vi "Station References Global.vi"() -> ()   [LabVIEW 2018]
panel:
  in  "Run Cal Popup":bool
  out "Oven_RTL":bool
  out "DMM3_RTL":bool
  out "DMM2_RTL":bool
  out "DMM1_RTL":bool
  out "PS3_RTL":bool
  out "PS2_RTL":bool
  out "PS1_RTL":bool
  out "RF Switch_RTL":bool
  out "NFA_RTL":bool
  out "SigGen3_RTL":bool
  out "SigGen2_RTL":bool
  out "SigGen1_RTL":bool
  out "SA_RTL":bool
  out "PNA_RTL":bool
  out "VNA_RTL":bool
  in  "Gantry":refnum<visa-resource-name>="GPIB0::9::INSTR"
  out "Gantry Model":string
  out "Gantry Present?":bool
  in  "RF Switch":refnum<visa-resource-name>="GPIB0::9::INSTR"
  out "RF Switch Model":string
  out "RF Switch Present?":bool
  out "PNA Model":string
  in  "PNA":refnum<visa-resource-name>
  out "PNA Present?":bool
  out "TempSense1":tag
  out "TempSense1 Model":string
  out "TempSense1 Present?":bool
  in  "USBSigGen1 Device ID":refnum<visa-resource-name>
  out "USBSigGen1 Model":string
  out "USBSigGen1 Present?":bool
  out "DMM3 Model":string
  out "DMM3 Present?":bool
  in  "DMM3":refnum<visa-resource-name>="GPIB0::9::INSTR"
  out "DMM2 Model":string
  out "DMM2 Present?":bool
  in  "DMM2":refnum<visa-resource-name>="GPIB0::9::INSTR"
  out "NFA Model":string
  out "DMM1 Model":string
  out "Oven Model":string
  out "Test Station Information":string
  out "SigGen3 Model":string
  in  "SigGen3":refnum<visa-resource-name>
  out "Sig Gen3 Present?":bool
  out "DMM1 Present?":bool
  in  "DMM1":refnum<visa-resource-name>="GPIB0::9::INSTR"
  out "NFA Present?":bool
  in  "NFA":refnum<visa-resource-name>="GPIB0::8::INSTR"
  out "Oven Present?":bool
  in  "Oven":refnum<visa-resource-name>
  out "VNA Present?":bool
  out "VNA Model":string
  in  "VNA":refnum<visa-resource-name>
  out "SigGen2 Model":string
  out "SigGen1 Model":string
  out "Spectrum Analyzer Model":string
  out "PS3 Model":string
  out "PS2 Model":string
  out "PS1 Model":string
  out "NI DAQ Present?":bool
  in  "NI DAQ":tag
  out "Sig Gen2 Present?":bool
  out "Sig Gen1 Present?":bool
  out "PS3 Present?":bool
  out "PS2 Present?":bool
  out "PS1 Present?":bool
  out "Spectrum Analyzer Present?":bool
  in  "PS2":refnum<visa-resource-name>
  in  "PS3":refnum<visa-resource-name>
  in  "PS1":refnum<visa-resource-name>
  in  "Spectrum Analyzer":refnum<visa-resource-name>
  in  "SigGen1":refnum<visa-resource-name>
  in  "SigGen2":refnum<visa-resource-name>
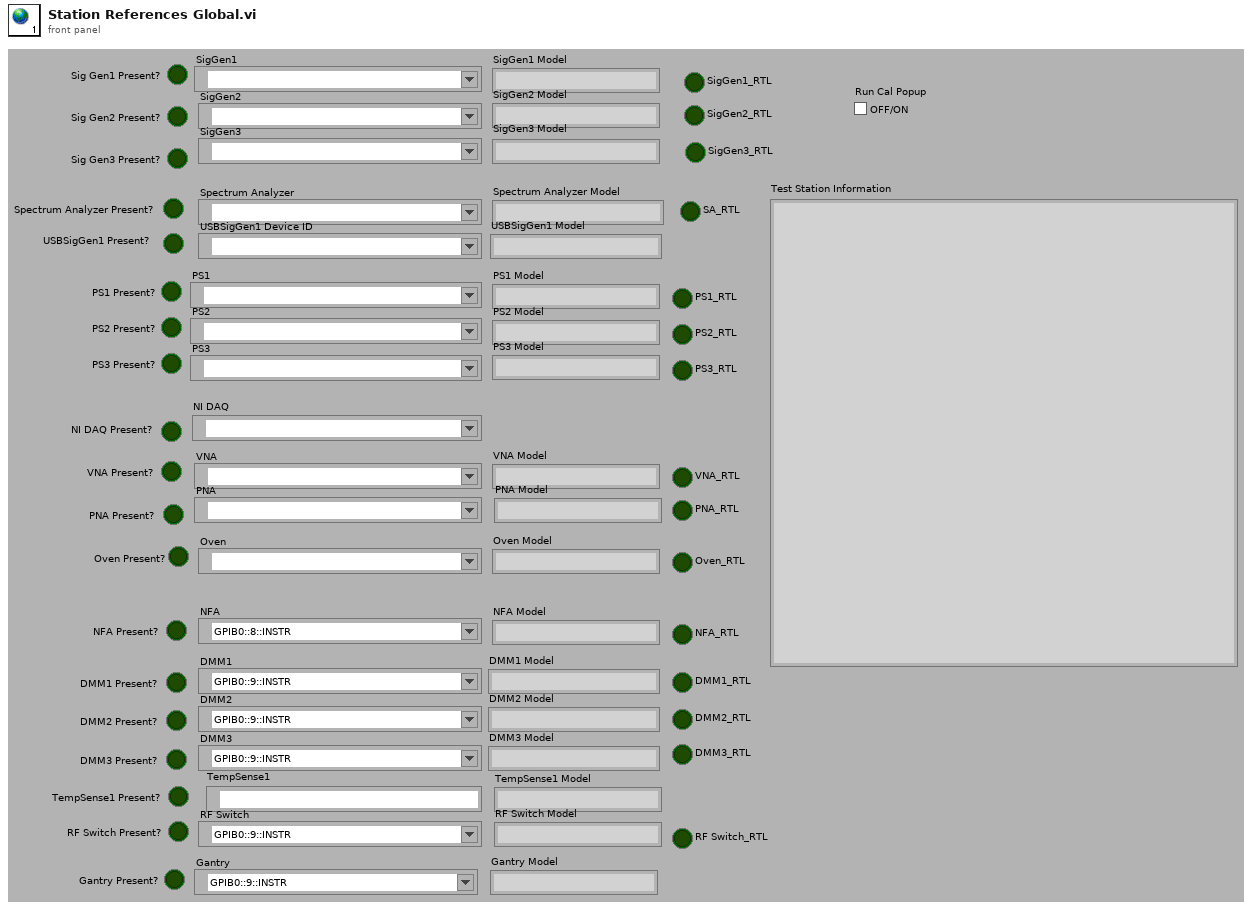
[diagram p1: front panel]
diagram:
